vi "23384_Davis_Poku_Amankwa_Amankwa.DavisPoku.MNE1201.1.6_348252_578184843.vi"() -> ()   [LabVIEW 2018]
panel:
  out "Parity":string
  in  "integer":dbl
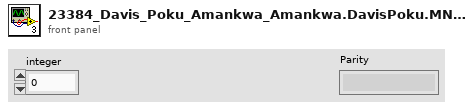
[diagram p1: front panel]
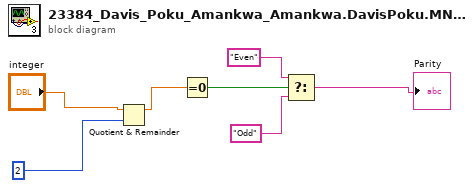
[diagram p0: block diagram]
diagram:
  n1 = Quotient & Remainder(x="integer", y=2) -> (x-y*floor(x/y)=w3:dbl)  [unwired: 1 out]
  n2 = Equal To 0?(x=w3) -> (x = 0?=w6:bool)
  n3 = Select(t="Even", s=w6, f="Odd") -> (s? t:f=→"Parity":string)
